vi "FTW-Subscription-Construct.vi"(5 "Publisher Address":string="tcp://127.0.0.1:5555", 7 "Topic":string, 11 "error in":errorcluster) -> (4 "FTW Subscription":refnum<class "FTW-Subscription.lvclass">, 6 "Incoming Message":refnum<event-registration>, 15 "error out":errorcluster)   [LabVIEW 2013, in "FTW-Subscription.lvclass"]
uses:
  FTW-Subscription.lvclass
  socket/FTW-Socket.lvclass
  socket/FTW-Socket-Type.ctl
panel:
  # "Inputs"
  # "Outputs"
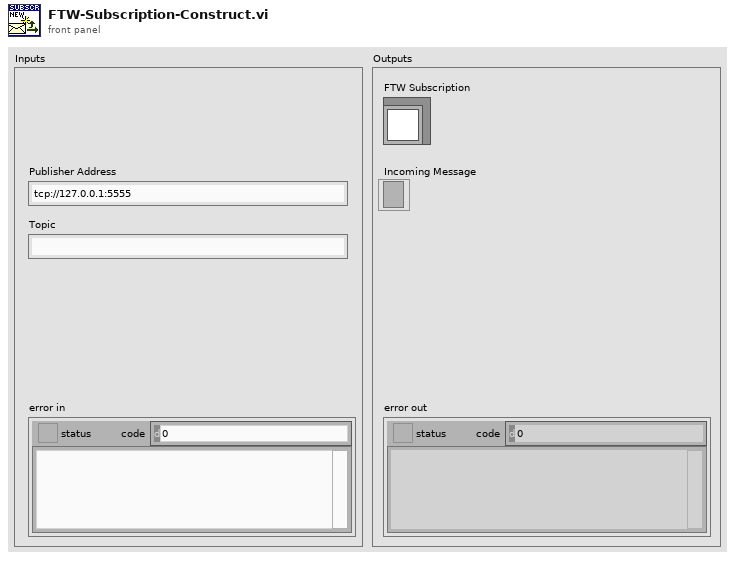
[diagram p1: front panel]
types:
  T1 = typedef "FTW-Socket.lvclass/FTW-Socket-Type.ctl" = enum32{"Server", "Client", "Publisher", "Subscriber", "Pipeline Producer", "Pipeline Consumer", "Surveyor", "Respondent", "Exclusive Pair", "Bus"}
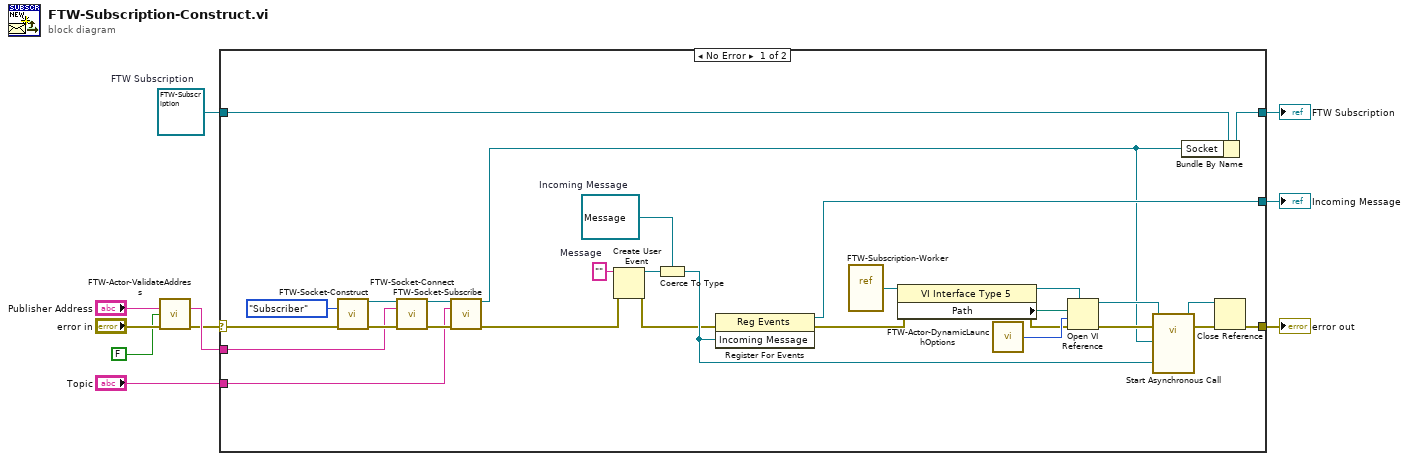
[diagram p0: block diagram]
diagram:
  w8 = refnum<class "FTW-Subscription.lvclass"> refnum  # FTW Subscription
  n1 = call "FTW-Actor-ValidateAddress.vi"("Address"="Publisher Address", "Allow wildcard replacement?"=FALSE, "error in"="error in") -> ("Sanitized Address"=w6:string, "error out"=w4:errorcluster)  [unwired: 10 in, 1 out]
  n2 = case shown="No Error" w4 {
    selector: w4 -> [w21 w41]
    tunnel: [w38 w40] -> w10
    tunnel: [w23 w41] -> w9
    tunnel: w8 -> [w39 w40]
    tunnel: w6 -> [w16 _]
    tunnel: [w19 _] -> w2
    tunnel: "Topic" -> [w11 _]
    frame No Error {
      w20 = ""  # Message
      w33 = refnum<user-event> refnum  # Incoming Message
      n3 = call "FTW-Socket-Construct.vi"("Socket Topology"=FTW-Socket-Type."Subscriber", "error in"=w21) -> ("FTW Socket"=w18:refnum<class "FTW-Socket.lvclass">, "error out"=w17:errorcluster)  [unwired: 12 in]
      n4 = call "FTW-Socket-Connect.vi"("FTW Socket"=w18, "Remote Address"=w16, "error in"=w17) -> ("FTW Socket out"=w14:refnum<class "FTW-Socket.lvclass">, "error out"=w13:errorcluster)  [unwired: 11 in]
      n5 = call "FTW-Socket-Subscribe.vi"("FTW Socket"=w14, "Topic"=w11, "error in"=w13) -> ("FTW Socket out"=w15:refnum<class "FTW-Socket.lvclass">, "error out"=w12:errorcluster)  [unwired: 11 in]
      n6 = Create User Event(user event datatype=w20, error in=w12) -> (user event=w32:refnum<user-event>, error out=w31:errorcluster)
      n7 = Coerce To Type(0:w32, 1:w33) -> (2:w37:refnum<user-event>)
      n8 = register-events(error in=w31, w37) -> (reference out=w19:refnum<event-registration>, error out=w34:errorcluster)  [unwired: 1 in]
      n9 = vi-ref "FTW-Subscription-Worker.vi"() -> (w24:refnum<vi>)
      n10 = property class="VI Interface Type 5"(reference=w24, error in=w34) -> (reference out=w25:refnum<vi>, error out=w28:errorcluster, "Path"=w26:path)
      n11 = call "FTW-Actor-DynamicLaunchOptions.vi"() -> ("Open VI Ref Options"=w29:i32)  [unwired: 1 in]
      n12 = Open VI Reference(type specifier VI Refnum (for type only)=w25, vi path=w26, options=w29, error in (no error)=w28) -> (vi reference=w30:refnum<vi>, error out=w27:errorcluster)  [unwired: 2 in]
      n13 = call-by-ref "Start Asynchronous Call"(reference=w30, error in=w27, "Backend Handler"=w37, "SubscriptionID"=w15) -> (reference out=w35:refnum<vi>, error out=w36:errorcluster)  [unwired: 1 in]
      n14 = Bundle By Name(cluster=w39, "Socket"=w15) -> (w38:refnum<class "FTW-Subscription.lvclass">)
      n15 = Close Reference(reference=w35, error in (no error)=w36) -> (error out=w23:errorcluster)
    }
    frame Error {
    }
  }
  "error out" <- w9
  "FTW Subscription" <- w10
  "Incoming Message" <- w2
